vi "GetDiagramInputs.vi"(6 "error in":errorcluster, 9 "ForLoop in":refnum<class "ForLoop.lvclass">) -> (0 "error out":errorcluster, 3 "ForLoop out":refnum<class "ForLoop.lvclass">, 4 "inputs terminals":refnum<class "Terminal.lvclass">[][](array[class]))   [LabVIEW 2014, in "Raspberry Pi Compatible Compiler for LabVIEW.lvlib" / "ForLoop.lvclass"]
uses:
  ForLoop.lvclass
  Terminal/Terminal.lvclass
  ForLoop.lvclass/ForLoop.ctl
  Tunnel/Tunnel.lvclass/Tunnel.ctl
  Loop/Loop.lvclass
  Tunnel/Tunnel.lvclass
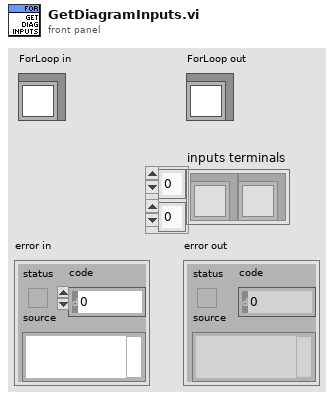
[diagram p1: front panel]
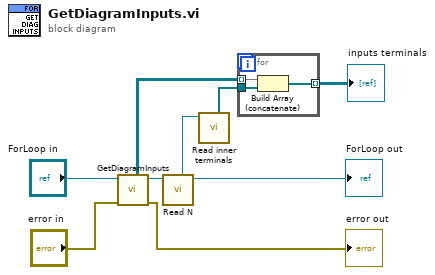
[diagram p0: block diagram]
diagram:
  n1 = call-parent "GetDiagramInputs.vi"("error in"="error in", "Loop in"="ForLoop in") -> ("error out"=→"error out":errorcluster, "Loop out"=w7:refnum<class "ForLoop.lvclass">, "inputs terminals"=w4:refnum<class "Terminal.lvclass">[][])  [unwired: 5 in]
  n2 = call "Read N.vi"("ForLoop in"=w7) -> ("ForLoop out"=→"ForLoop out":refnum<class "ForLoop.lvclass">, "N"=w2:refnum<class "Tunnel.lvclass">)  [unwired: 7 in]
  n3 = call "Read inner terminals.vi"("Tunnel in"=w2) -> ("inner terminals"=w1:refnum<class "Terminal.lvclass">[])  [unwired: 7 in, 1 out]
  n4 = for {
    tunnel: w1 -> [w12]
    tunnel: w4 -> [w11] mode=indexing
    tunnel: [w10] -> w3 mode=indexing
    n5 = Build Array (concatenate)(w11, w12) -> (w10:refnum<class "Terminal.lvclass">[])
  }
  "inputs terminals" <- w3
